vi "Memory manager V5 with delay.vi"   [LabVIEW 2015]
uses:
  <vilib>/Platform/TimedLoop/XDataNode/timing_clust.ctl
  <vilib>/Platform/TimedLoop/XDataNode/nitl_modes.ctl
  <vilib>/Platform/TimedLoop/XDataNode/wakeup.ctl
  <vilib>/rvi/Emulation/niFpgaSctlEmulationGetInTimedLoop.vi
  <vilib>/rvi/Emulation/niFpgaEmulationReportErrorSimple.vi
  <vilib>/rvi/Emulation/niFpgaGetClockAttributes.vi
  <vilib>/rvi/Emulation/niFpgaCriticalErrorInLSC.vi
  LIDAR Slave Globals.vi
  <vilib>/rvi/Emulation/niFpgaEmulationIsFPGAContextNoSignature.vi
  <vilib>/rvi/errors/niFpgaSetErrorForExecOnDevCompSimple.vi
  <vilib>/rvi/eio/common/nirviEmuReportErrorAndStop.vi
  <vilib>/rvi/DataTransferAndStorage/Container/Common/niFpgaContainerGetUniqueNameForEmu.vi
  <vilib>/rvi/FIFO/Fifo_Resource/nirvififoEmulationSetSize.vi
  <vilib>/rvi/FIFO/Fifo_Resource/nirviFifoEmulationQueueMgr.vi
  <instcachedir>/0/nirviFifoEmulationQueueMgr_E5CAEC123FF24DC58D834DCA3CDAA9B5.lvgen/nirviFifoEmulationQueueMgr_E5CAEC123FF24DC58D834DCA3CDAA9B5_000.vi
  <vilib>/Utility/error.llb/Clear Errors.vi
  <vilib>/rvi/FIFO/Fifo_Resource/nirvififoEmulationCreateLock.vi
  <vilib>/rvi/Emulation/niFpgaProcessEmulError.vi
  <vilib>/rvi/FIFO/Fifo_Resource/nirvififoEmulationObtainLock.vi
  <vilib>/rvi/FIFO/Fifo_Resource/nirvififoEmulationReleaseLock.vi
  <vilib>/rvi/occurrence/nirviWaitOnOccurrenceBase.vi
  <vilib>/rvi/errors/nirviReportUnexpectedCaseInternalError.vi
  <vilib>/rvi/errors/nirviReportUnexpectedCaseInternalError (U32).vi
  <vilib>/rvi/Memory/Memory_Emulation/nirvimemoryFastEmulation.vi
  <vilib>/rvi/Memory/Memory_Emulation/nirvimemoryEmulation.vi
  <vilib>/rvi/FIFO/Fifo_Resource/nirvififoEmulationDetermineInputValidOut.vi
  <vilib>/Platform/TimedLoop/XDataNode/XDataNode.xnode
  <vilib>/rvi/DataTransferAndStorage/Container/XNode/niFpgaContainer.xnode
  <vilib>/rvi/FIFO/Fifo_Resource/nirvififoEmulationRead.vi
  <vilib>/rvi/FIFO/Fifo_Resource/nirvififoEmulationWrite.vi
  <vilib>/rvi/FXPMathLib/FxpAdd/XNode/nifxpmath_Add.xnode
  <vilib>/Platform/TimedLoop/XDataNode/XDNodeRunTimeDep.lvlib
  <vilib>/rvi/FXPMathLib/sim/FxpSim.dll
types:
  T1 = typedef "XDNodeRunTimeDep.lvlib/timing_clust.ctl" = cluster{"Expected End [f-1]":u64, "Actual End [f-1]":u64, "Finished Late? [f-1]":bool, "Expected End [i-1]":u64, "Actual End [i-1]":u64, "Finished Late? [i-1]":bool, "Expected Start [i]":u64, "Actual Start [i]":u64, "Expected Start [f]":u64, "Actual Start [f]":u64, "Source Name":string, "Structure Name":string, "Period":i64, "Deadline":i64, "Offset":i64, "Start":i64, "Priority":i32, "Timeout":i32, "Mode":T2, "Wakeup Reason":T3, "Error":errorcluster, "Source Type":string, "Secondary Source Type":string, "Global End Time":u64, "Global Start Time":u64, "Frame Duration":u64, "Iteration Duration":u64, "Assigned CPU":i32, "I/O Scan Engine Mode":u32}
  T2 = typedef "XDNodeRunTimeDep.lvlib/nitl_modes.ctl" = enum32{"No Change", "Process missed periods, maintain original phase", "Discard missed periods, maintain original phase", "Process missed periods, ignore original phase", "Discard missed periods, ignore original phase"}
  T3 = typedef "XDNodeRunTimeDep.lvlib/wakeup.ctl" = enum32{"Normal", "Aborted", "Asynchronous wakeup", "Timing source error", "Timed loop error", "Timeout"}
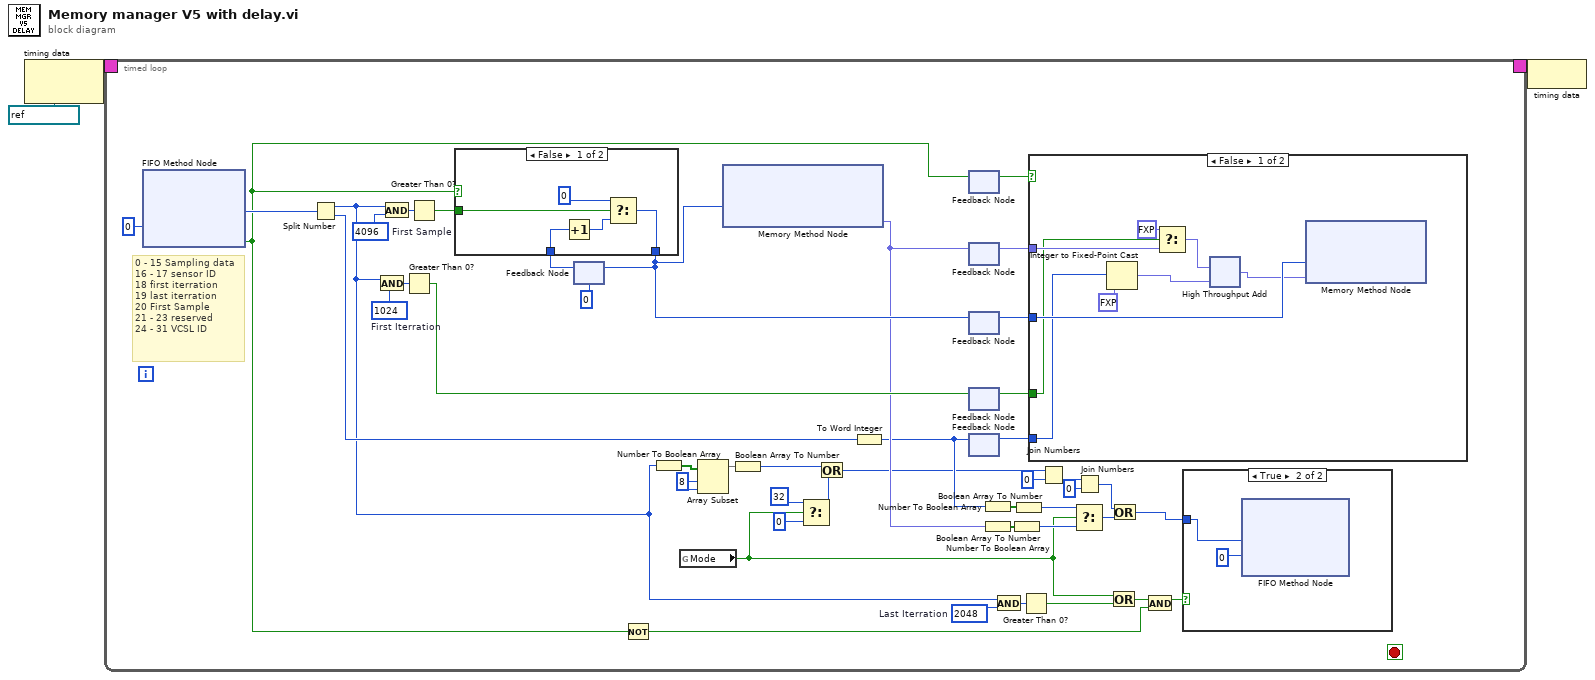
[diagram p0: block diagram]
diagram:
  n1 = node-c288(refnum<k21> "130MHz" ("Source Name")) -> (w3:T1)
  n2 = timed-loop {
    timing: w3 -> [_]
    timing-out: [_] -> w2
    stop <- _ stop-if-true
    w17 = 8 ("index")
    w36 = u16 1024  # First Iterration
    w42 = u16 2048  # Last Iterration
    w45 = u16 4096  # First Sample
    # "0 - 15 Sampling data\n16 - 17 sensor ID\n18 first iterration\n19 last iterration\n20 First Sample\n21 - 23 reserved\n24 - 31 VCSL ID"
    n3 = xnode ("FIFO Method Node")("Timeout"=0) -> ("Element"=w33:u32, "Timed Out?"=w32:bool)  [unwired: 1 in, 1 out]
    n4 = Split Number(x=w33) -> (hi(x)=w18:u16, lo(x)=w44:u16)
    n5 = And(x=w18, y=w36) -> (x .and. y?=w37:u16)
    n6 = And(x=w18, y=w45) -> (x .and. y?=w46:u16)
    n7 = Greater Than 0?(x=w37) -> (x > 0?=w34:bool)
    n8 = Greater Than 0?(x=w46) -> (x > 0?=w35:bool)
    n9 = feedback #1(u32 0 ("Element")) -> (w47:u32)
    n10 = case shown="False" w32 {
      tunnel: [w64 w66] -> w31
      tunnel: w47 -> [w63 w66]
      tunnel: w35 -> [w61 _]
      frame False {
        n11 = Increment(x=w63) -> (x+1=w62:u32)
        n12 = Select(t=u32 0 ("Element"), s=w61, f=w62) -> (s? t:f=w64:u32)
      }
      frame True {
      }
    }
    n13 = feedback-in #1(w31) -> ()
    n14 = Not(x=w32) -> (.not. x?=w38:bool)
    n15 = Number To Boolean Array(number=w18) -> (Boolean array=w16:bool[])
    n16 = global read "LIDAR Slave Globals.vi" "Mode"() -> (w9:bool)
    n17 = Array Subset(array=w16, index=w17, length=w17) -> (w15:bool[])
    n18 = xnode ("Memory Method Node")("Address"=w31) -> ("Data"=w26:fxp<+/-,22,22>)  [unwired: 1 in, 1 out]
    n19 = Boolean Array To Number(Boolean array=w15) -> (number=w14:u8)
    n20 = Select(t=u8 32 ("y"), s=w9, f=u8 0) -> (s? t:f=w11:u8)
    n21 = Or(x=w14, y=w11) -> (x .or. y?=w13:u8)
    n22 = To Word Integer(number=w44) -> (16bit integer=w25:i16)
    n23 = feedback-in #2(w32) -> ()
    n24 = feedback #2() -> (w8:bool)  [unwired: 1 in]
    n25 = feedback-in #3(w26) -> ()
    n26 = feedback #3() -> (w7:fxp<+/-,22,22>)  [unwired: 1 in]
    n27 = feedback-in #4(w31) -> ()
    n28 = feedback #4() -> (w6:u32)  [unwired: 1 in]
    n29 = feedback-in #5(w34) -> ()
    n30 = feedback #5() -> (w5:bool)  [unwired: 1 in]
    n31 = feedback-in #6(w25) -> ()
    n32 = feedback #6() -> (w4:i16)  [unwired: 1 in]
    n33 = Number To Boolean Array(number=w25) -> (Boolean array=w29:bool[])
    n34 = Number To Boolean Array(number=w26) -> (Boolean array=w27:bool[])
    n35 = And(x=w18, y=w42) -> (x .and. y?=w43:u16)
    n36 = Boolean Array To Number(Boolean array=w27) -> (number=w28:u32)
    n37 = Boolean Array To Number(Boolean array=w29) -> (number=w30:u32)
    n38 = Greater Than 0?(x=w43) -> (x > 0?=w41:bool)
    n39 = case shown="False" w8 {
      tunnel: w7 -> [w59 _]
      tunnel: w4 -> [w52 _]
      tunnel: w6 -> [w57 _]
      tunnel: w5 -> [w53 _]
      frame False {
        n40 = Integer to Fixed-Point Cast(fixed-point type=fxp<+/-,16,16> 0.0, integer=w52) -> (fixed-point=w54:fxp<+/-,16,16>)
        n41 = Select(t=fxp<+/-,22,22> 0.0, s=w53, f=w59) -> (s? t:f=w58:fxp<+/-,22,22>)
        n42 = xnode ("High Throughput Add")("x"=w58, "y"=w54) -> ("x+y"=w56:fxp<+/-,22,22>)
        n43 = xnode ("Memory Method Node")("Address"=w57, "Data"=w56) -> ()  [unwired: 1 in, 1 out]
      }
      frame True {
      }
    }
    n44 = Join Numbers(hi=w13, lo=u8 0) -> ((hi.lo)=w23:u16)
    n45 = Select(t=w30, s=w9, f=w28) -> (s? t:f=w21:u32)
    n46 = Join Numbers(hi=w23, lo=u16 0) -> ((hi.lo)=w20:u32)
    n47 = Or(x=w9, y=w41) -> (x .or. y?=w40:bool)
    n48 = Or(x=w20, y=w21) -> (x .or. y?=w19:u32)
    n49 = And(x=w40, y=w38) -> (x .and. y?=w39:bool)
    n50 = case shown="True" w39 {
      tunnel: w19 -> [_ w50]
      frame False {
      }
      frame True {
        n51 = xnode ("FIFO Method Node")("Element"=w50, "Timeout"=0) -> ()  [unwired: 1 in, 2 out]
      }
    }
  }
  n52 = node-c288(w2) -> ()
